vi "Do.vi"(8 "error in (no error)":errorcluster, 10 "Msg Queue":refnum<queue>, 11 "State Cmd in":refnum<class "Exe Msg.lvclass">=refnum) -> (0 "error out":errorcluster, 3 "State Cmd out":refnum<class "Exe Msg.lvclass">)   [LabVIEW 2020, in "OOP SM.lvlib" / "Exe Msg.lvclass"]
uses:
  Exe Msg.lvclass
  E:/NI I Program/Actor Intr Demo/OOP SM/Message/Message.lvclass
  Message/Message.lvclass
  OOP SM.lvlib
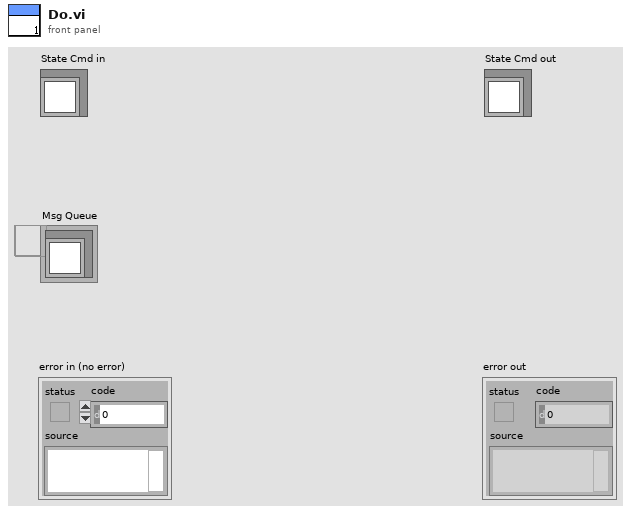
[diagram p1: front panel]
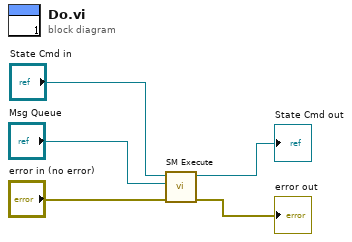
[diagram p0: block diagram]
diagram:
  n1 = call "SM Execute.vi"("error in (no error)"="error in (no error)", "Msg Queue"="Msg Queue", "Message in"="State Cmd in") -> ("error out"=→"error out":errorcluster, "Message out"=→"State Cmd out":refnum<class "Exe Msg.lvclass">)  [unwired: 7 in]
